vi "relay-sample.vi"   [LabVIEW 2020]
uses:
  <vilib>/Rock Robotics/SystemInterfaces/DIO/FPGA_DIORelayChannel.ctl
  <vilib>/Rock Robotics/WPI/Relay/WPI_RelayDirection.ctl
types:
  T1 = typedef "WPI_RelayDirection.ctl" = enum16{"Both directions", "Forward only", "Reverse only"}
  T2 = typedef "FPGA_DIORelayChannel.ctl" = enum8{"Relay 0", "Relay 1", "Relay 2", "Relay 3", "Invalid"}
  T3 = typedef "WPI_RelayDevRef.ctl" = cluster{"DevStatus":errorcluster, "Relay Channel":T2, "Relay Direction":T1}
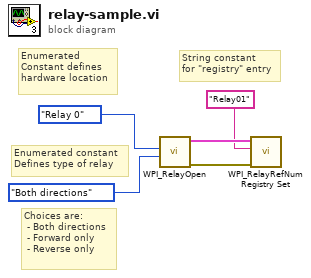
[diagram p0: block diagram]
diagram:
  # "Choices are:\n - Both directions\n - Forward only\n - Reverse only"
  # "String constant\nfor \"registry\" entry"
  # "Enumerated constant\nDefines type of relay"
  # "Enumerated\nConstant defines\nhardware location"
  n1 = call <vilib>:"WPI_RelayOpen.vi"("Relay Direction"=WPI_RelayDirection."Both directions", "Relay Channel"=FPGA_DIORelayChannel."Relay 0") -> ("error out"=w1:errorcluster, "RelayDevRef"=w5:T3)  [unwired: 8 in]
  n2 = call <vilib>:"WPI_RelayRefNum Registry Set.vi"("error in (no error)"=w1, "refnum name"="Relay01", "RelayDevRef"=w5) -> ()  [unwired: 7 in, 2 out]
